vi "Limelight Tag Distances.vi"() -> (1 "Front":dbl, 2 "Right":dbl, 3 "Left":dbl)   [LabVIEW 2025]
uses:
  <vilib>/Rock Robotics/Network Tables/NT Read Numeric Array.vi
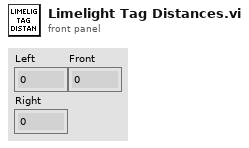
[diagram p1: front panel]
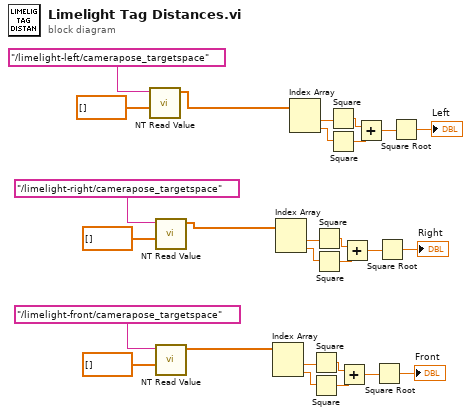
[diagram p0: block diagram]
diagram:
  n1 = call-poly <vilib>:"NT Read Value.vi"("default value"=dbl[] [], "name"="/limelight-left/camerapose_targetspace") -> ("value"=w21:dbl[])  [unwired: 7 in, 2 out]
  n2 = call-poly <vilib>:"NT Read Value.vi"("default value"=dbl[] [], "name"="/limelight-right/camerapose_targetspace") -> ("value"=w8:dbl[])  [unwired: 7 in, 2 out]
  n3 = call-poly <vilib>:"NT Read Value.vi"("default value"=dbl[] [], "name"="/limelight-front/camerapose_targetspace") -> ("value"=w1:dbl[])  [unwired: 7 in, 2 out]
  n4 = Index Array(array=w1) -> (element #1=w7:dbl, element #2=w6:dbl)  [unwired: 2 in]
  n5 = Index Array(array=w8) -> (element #1=w9:dbl, element #2=w10:dbl)  [unwired: 2 in]
  n6 = Index Array(array=w21) -> (element #1=w20:dbl, element #2=w19:dbl)  [unwired: 2 in]
  n7 = Square(x=w7) -> (x^2=w5:dbl)
  n8 = Square(x=w6) -> (x^2=w4:dbl)
  n9 = Square(x=w9) -> (x^2=w11:dbl)
  n10 = Square(x=w10) -> (x^2=w12:dbl)
  n11 = Square(x=w20) -> (x^2=w18:dbl)
  n12 = Square(x=w19) -> (x^2=w17:dbl)
  n13 = Add(x=w5, y=w4) -> (x+y=w3:dbl)
  n14 = Add(x=w11, y=w12) -> (x+y=w13:dbl)
  n15 = Add(x=w18, y=w17) -> (x+y=w16:dbl)
  n16 = Square Root(x=w3) -> (sqrt(x)=→"Front":dbl)
  n17 = Square Root(x=w13) -> (sqrt(x)=→"Right":dbl)
  n18 = Square Root(x=w16) -> (sqrt(x)=→"Left":dbl)
